vi "To String (Object).vi"(6 "pretty print? (T)":bool=TRUE, 7 "enable LabVIEW extensions? (T)":bool=TRUE, 8 "error in (no error)":errorcluster, 10 "indent":i32, 11 "JSON Value in":variant) -> (0 "error out":errorcluster, 3 "String":string)   [LabVIEW 2017, in "Advanced Variant Tools.lvlib"]
doc: "Flattens the given JSON data to a string."
uses:
  Advanced Variant Tools.lvlib
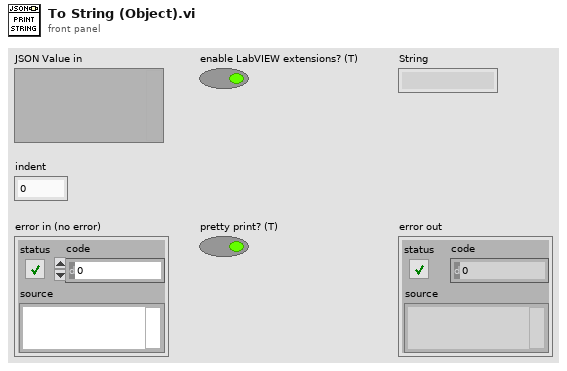
[diagram p1: front panel]
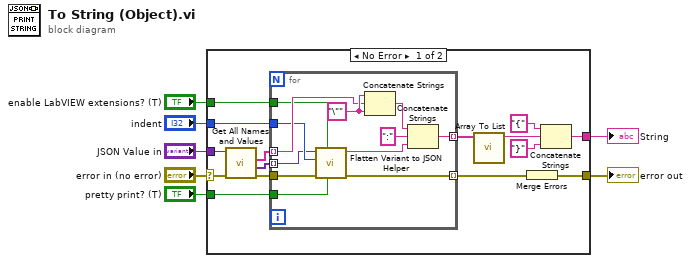
[diagram p0: block diagram]
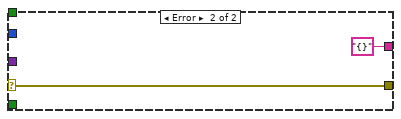
[diagram p2: hidden frame]
diagram:
  n1 = case shown="No Error" "error in (no error)" {
    selector: "error in (no error)" -> [w11 w35]
    tunnel: "JSON Value in" -> [w12 _]
    tunnel: [w22 "{}"] -> w6
    tunnel: [w18 w35] -> w4
    tunnel: "enable LabVIEW extensions? (T)" -> [w15 _]
    tunnel: "indent" -> [w14 _]
    tunnel: "pretty print? (T)" -> [w10 _]
    frame No Error {
      n2 = call "Get All Names and Values.vi"("error in"=w11, "Variant (Cluster) In"=w12) -> ("error out"=w9:errorcluster, "Values"=w8:variant[], "Item Names"=w13:string[])  [unwired: 5 in, 2 out]
      n3 = for {
        tunnel: w13 -> [w31] mode=indexing
        tunnel: w8 -> [w23] mode=indexing
        tunnel: [w33] -> w21 mode=indexing
        tunnel: w9 -> [w24]
        tunnel: [w28] -> w19 mode=indexing
        tunnel: w15 -> [w27]
        tunnel: w14 -> [w26]
        tunnel: w10 -> [w25]
        w32 = "\"" ("string")
        n4 = call "Flatten Variant to JSON Helper.vi"("pretty print? (T)"=w25, "enable LabVIEW extensions? (T)"=w27, "error in (no error)"=w24, "indent"=w26, "JSON Value in"=w23) -> ("error out"=w28:errorcluster, "String"=w29:string)  [unwired: 5 in]
        n5 = Concatenate Strings(w32, w31, w32) -> (w30:string)
        n6 = Concatenate Strings(w30, ":" ("string"), w29) -> (w33:string)
      }
      n7 = call "Array To List.vi"("Array"=w21) -> ("String"=w20:string)  [unwired: 10 in]
      n8 = Merge Errors(w19) -> (w18:errorcluster)
      n9 = Concatenate Strings("{" ("string"), w20, "}" ("string")) -> (w22:string)
    }
    frame Error {
    }
  }
  "String" <- w6
  "error out" <- w4
